vi "Rx Stream control.vi"(0 "data in":T1[](array[typedef]), 9 "input valid":bool, 11 "niUSRP Rx Core v1 FPGA.lvclass":refnum<class "niUSRP Sync v1 FPGA.lvclass">, 12 "ready for output":bool) -> (4 "data out":T1[](array[typedef]), 10 "output valid":bool, 14 "ready for input":bool, 15 "niUSRP Rx Core v1 FPGA.lvclass 2":refnum<class "niUSRP Sync v1 FPGA.lvclass">)   [LabVIEW 2025, in "niUSRP Sync v1 FPGA.lvclass"]
uses:
  niUSRP Rx Core v1 FPGA/niUSRP Sync v1 FPGA.lvclass
  niUSRP Rx Core v1 FPGA/niUSRP Sync v1 FPGA.lvclass/niUSRP Sync v1 FPGA.ctl
  <instrlib>/_niInstr/Basic Elements/v1/FPGA/niInstr Basic Elements v1 FPGA.lvlib
  <vilib>/rvi/DataTransferAndStorage/Container/XNode/niFpgaContainer.xnode
  <vilib>/rvi/DataTransferAndStorage/Register/Emulation/niFpgaRegisterEmulationRefIn.vi
  <instrlib>/_niInstr/DSP/v1/Shared/Public/IQ Data.ctl
  <instrlib>/_niInstr/DSP/v1/Shared/niInstr DSP v1 Shared.lvlib
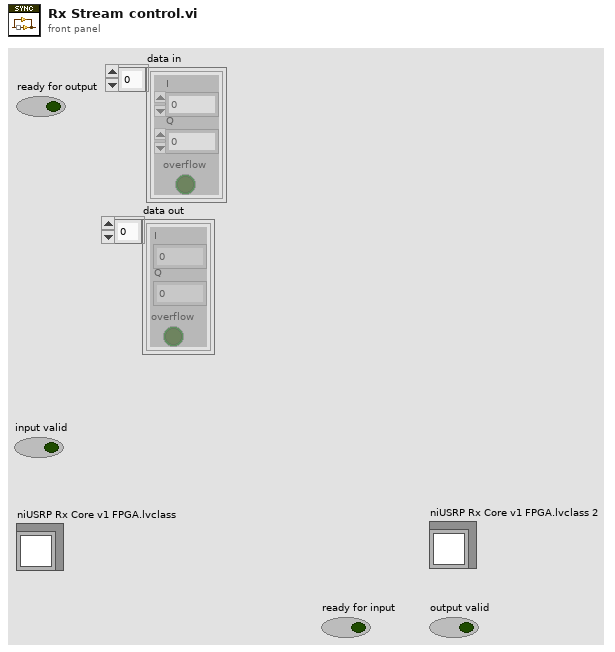
[diagram p1: front panel]
types:
  T1 = typedef "niInstr DSP v1 Shared.lvlib/IQ Data.ctl" = cluster{"I":fxp<+/-,18,1>, "Q":fxp<+/-,18,1>, "overflow":bool}
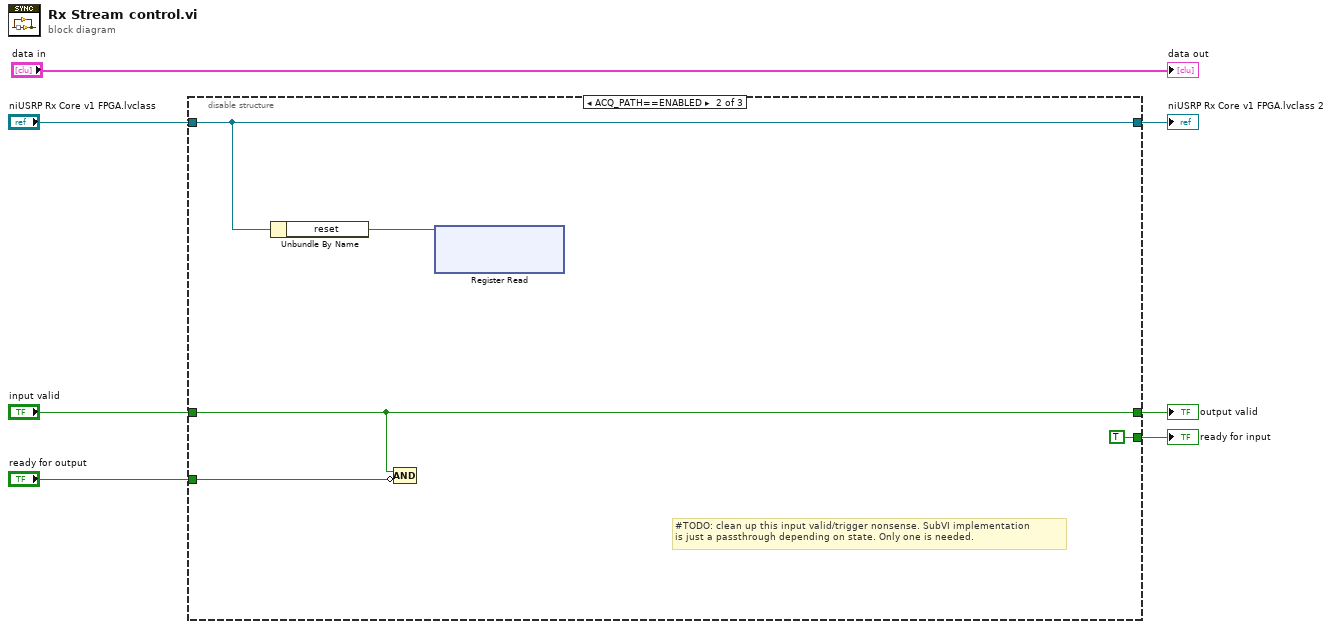
[diagram p0: block diagram]
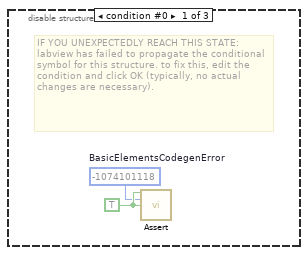
[diagram p2: hidden frame]
diagram:
  n1 = disable-structure shown="ACQ_PATH==ENABLED" {
    disable-tunnel: "input valid" -> [_ w11 _]
    disable-tunnel: "niUSRP Rx Core v1 FPGA.lvclass" -> [_ w12 _]
    disable-tunnel: "ready for output" -> [_ w13 _]
    disable-tunnel: [_ w12 _] -> w4
    disable-tunnel: [_ w11 _] -> w2
    disable-tunnel: [_ TRUE _] -> w1
    frame condition #0 {
      w9 = TRUE ("assert")
      w8 = -1074101118  # BasicElementsCodegenError
      # "IF YOU UNEXPECTEDLY REACH THIS STATE:\nlabview has failed to propagate the conditional symbol for this structure. to fix this, edit the condition and click OK (typically, no actual changes are necessary)."
      n2 = call <instrlib>:"Assert.vi"("assert"=w9, "error code"=w8, "enable show error"=w9) -> ()  [unwired: 13 in]
    }
    frame condition #1 (active) {
      # "#TODO: clean up this input valid/trigger nonsense. SubVI implementation\nis just a passthrough depending on state. Only one is needed."
      n3 = Unbundle By Name(w12) -> ("reset"=w14:refnum<k21>)
      n4 = Compound Arithmetic op=AND(w11, invert w13) -> ()  [unwired: 1 out]
      n5 = xnode ("Register Read")("Register In"=w14) -> ()  [unwired: 2 out]
    }
    frame condition #2 {
    }
  }
  "niUSRP Rx Core v1 FPGA.lvclass 2" <- w4
  "output valid" <- w2
  "ready for input" <- w1
  "data out" <- "data in"
